vi "Define Customized Character (5X8).vi"(8 "error in (no error)":errorcluster, 9 "customized character pattern":bool[][](array[boolean]), 10 "customized character code in":u8, 11 "HD44780 in":refnum<class "HD44780.lvclass">) -> (0 "error out":errorcluster, 2 "customized character code out":u8, 3 "HD44780 out":refnum<class "HD44780.lvclass">)   [LabVIEW 2017, in "HD44780.lvclass"]
uses:
  HD44780.lvclass
  HD44780.lvclass/HD44780.ctl
  Common/HD44780 Common.lvlib
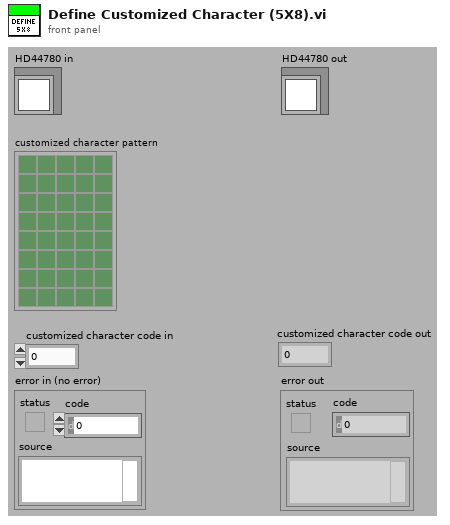
[diagram p1: front panel]
types:
  T1 = typedef "HD44780 Common.lvlib/cluster of class private data.ctl" = cluster{"FPGA VI Reference":refnum<k20>, "device index":i8, "screen size":T2, "font size":T3, "auto wrap":bool, "alignment":T4, "number of line":T5, "shift 0":i8, "entry mode 0":T6, "shift 1":i8, "entry mode 1":T6}
  T2 = typedef "HD44780 Common.lvlib/screen size.ctl" = enum8{"8x1", "8x2", "12x4", "16x1", "16x2", "16x4", "20x1", "20x2", "20x4", "24x1", "24x2", "40x2", "40x4"}
  T3 = typedef "HD44780 Common.lvlib/font size.ctl" = enum8{"5x8", "5x10"}
  T4 = typedef "HD44780 Common.lvlib/alignment.ctl" = enum16{"None", "Left", "Center", "Right"}
  T5 = typedef "HD44780 Common.lvlib/line number.ctl" = enum8{"1 line", "2 lines"}
  T6 = typedef "HD44780 Common.lvlib/entry mode.ctl" = enum8{"increment & no shift", "increment & shift", "decrement & no shift", "decrement & shift"}
  T7 = cluster{"FPGA VI Reference":refnum<k20>, "device index":i8, "screen size":enum8{"8x1", "8x2", "12x4", "16x1", "16x2", "16x4", "20x1", "20x2", "20x4", "24x1", "24x2", "40x2", "40x4"}, "font size":enum8{"5x8", "5x10"}, "auto wrap":bool, "alignment":enum16{"None", "Left", "Center", "Right"}, "number of line":enum8{"1 line", "2 lines"}, "shift 0":i8, "entry mode 0":enum8{"increment & no shift", "increment & shift", "decrement & no shift", "decrement & shift"}, "shift 1":i8, "entry mode 1":enum8{"increment & no shift", "increment & shift", "decrement & no shift", "decrement & shift"}}
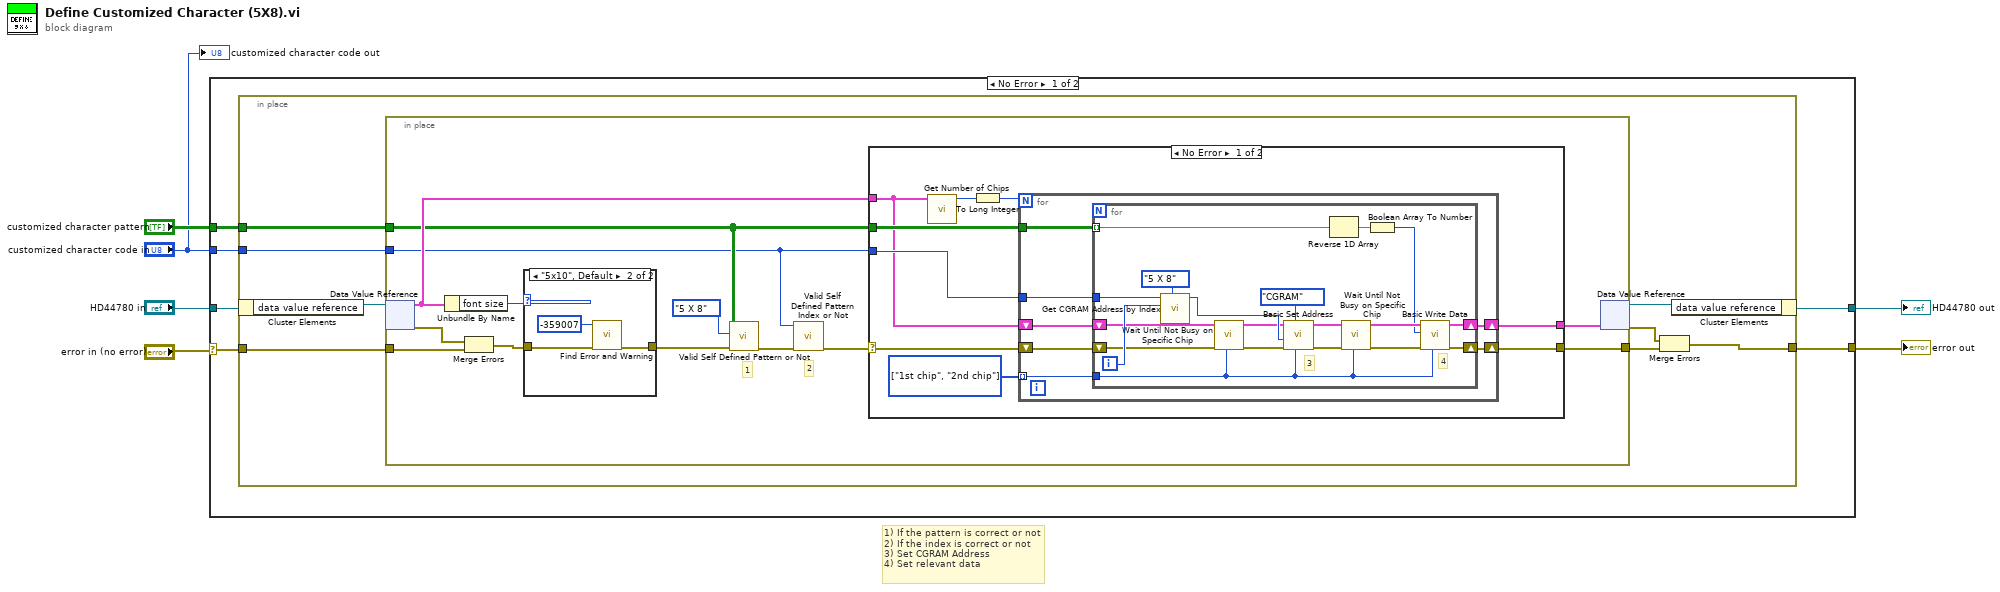
[diagram p0: block diagram]
diagram:
  # "1) If the pattern is correct or not\n2) If the index is correct or not\n3) Set CGRAM Address\n4) Set relevant data"
  n1 = case shown="No Error" "error in (no error)" {
    selector: "error in (no error)" -> [w11 w76]
    tunnel: [w12 w76] -> w5
    tunnel: [w9 w75] -> w3
    tunnel: "HD44780 in" -> [w10 w75]
    tunnel: "customized character pattern" -> [w8 _]
    tunnel: "customized character code in" -> [w7 _]
    frame No Error {
      n2 = in-place {
        in-place-border: [w13] -> w12
        in-place-border: w11 -> [w20]
        in-place-border: w8 -> [w17]
        in-place-border: w7 -> [w16]
        n3 = in-place-cluster #1(w10) -> ("data value reference"=w19:refnum<data-value>)
        n4 = in-place {
          in-place-border: [w33] -> w15
          in-place-border: w20 -> [w23]
          in-place-border: w17 -> [w25]
          in-place-border: w16 -> [w24]
          # "2"
          # "1"
          n5 = in-place-dvr #2(w19) -> (w29:T1, w26:errorcluster)
          n6 = Unbundle By Name(w29) -> ("font size"=w27:T3)
          n7 = Merge Errors(w26, w23) -> (w22:errorcluster)
          n8 = case shown="\"5x10\", Default" w27 {
            tunnel: [w34 w36] -> w28
            tunnel: w22 -> [w34 w35]
            frame "5x8" {
            }
            frame "5x10", Default {
              n9 = call "Find Error and Warning.vi"("error in (no error)"=w35, "error code"=-359007) -> ("error out"=w36:errorcluster)  [unwired: 9 in]
            }
          }
          n10 = call "Valid Self Defined Pattern or Not.vi"("error in (no error)"=w28, "self defined pattern"=enum16{"5 X 10", "5 X 8"}."5 X 8", "customized character pattern"=w25) -> ("error out"=w32:errorcluster)  [unwired: 8 in]
          n11 = call "Valid Self Defined Pattern Index or Not.vi"("error in (no error)"=w32, "customized character code"=w24) -> ("error out"=w31:errorcluster)  [unwired: 9 in]
          n12 = case shown="No Error" w31 {
            selector: w31 -> [w43 w74]
            tunnel: [w46 w74] -> w33
            tunnel: w25 -> [w42 _]
            tunnel: w24 -> [w41 _]
            tunnel: w29 -> [w40 w73]
            tunnel: [w38 w73] -> w21
            frame No Error {
              w44 = enum16{"1st chip", "2nd chip"}[] [enum."1st chip", enum."2nd chip"] items=["1st chip", "2nd chip"]
              n13 = call "Get Number of Chips.vi"("cluster of private data in"=w40) -> ("number of chips"=w45:u8)  [unwired: 10 in]
              n14 = To Long Integer(number=w45) -> (32bit integer=w39:i32)
              n15 = for {
                N: w39 -> [_]
                shift-right: [w53] -> w46
                shift-left: w43 -> [w52]
                tunnel: w44 -> [w50] mode=indexing
                tunnel: w42 -> [w48]
                tunnel: w41 -> [w51]
                shift-right: [w47] -> w38
                shift-left: w40 -> [w49]
                n16 = for {
                  shift-right: [w72] -> w53
                  shift-left: w52 -> [w62]
                  tunnel: w51 -> [w67]
                  tunnel: w50 -> [w60]
                  tunnel: w48 -> [w55] mode=indexing
                  shift-right: [w57] -> w47
                  shift-left: w49 -> [w59]
                  i -> [w65]
                  # "3"
                  # "4"
                  n17 = call "Get CGRAM Address by Index.vi"("self defined pattern"=enum16{"5 X 10", "5 X 8"}."5 X 8", "index of row"=w65, "customized character index"=w67) -> ("CGRAM address"=w66:u8)  [unwired: 8 in]
                  n18 = call "Wait Until Not Busy on Specific Chip.vi"("chip select  (1st chip)"=w60, "error in (no error)"=w62, "cluster of private data in"=w59) -> ("error out"=w61:errorcluster, "cluster of private data out"=w58:T7)  [unwired: 7 in]
                  n19 = call "Basic Set Address.vi"("chip select  (1st chip)"=w60, "address type (DDRAM)"=enum16{"DDRAM", "CGRAM"}."CGRAM" ("address type (DD RAM)"), "error in (no error)"=w61, "address (0, 0)"=w66, "cluster of private data in"=w58) -> ("error out"=w69:errorcluster, "cluster of private data out"=w64:T7)  [unwired: 5 in]
                  n20 = Reverse 1D Array(array=w55) -> (reversed array=w56:bool[])
                  n21 = call "Wait Until Not Busy on Specific Chip.vi"("chip select  (1st chip)"=w60, "error in (no error)"=w69, "cluster of private data in"=w64) -> ("error out"=w71:errorcluster, "cluster of private data out"=w63:T7)  [unwired: 7 in]
                  n22 = Boolean Array To Number(Boolean array=w56) -> (number=w54:u8)
                  n23 = call "Basic Write Data.vi"("chip select  (1st chip)"=w60, "error in (no error)"=w71, "character code"=w54, "cluster of private data in"=w63) -> ("error out"=w72:errorcluster, "cluster of private data out"=w57:T7)  [unwired: 6 in]
                }
              }
            }
            frame Error {
            }
          }
          n24 = in-place-dvr #2(w21) -> (w18:refnum<data-value>, w14:errorcluster)
        }
        n25 = Merge Errors(w14, w15) -> (w13:errorcluster)
        n26 = in-place-cluster #1("data value reference"=w18) -> (w9:refnum<class "HD44780.lvclass">)
      }
    }
    frame Error {
    }
  }
  "error out" <- w5
  "HD44780 out" <- w3
  "customized character code out" <- "customized character code in"
